vi "Voltage output module.vi"(0 "Device Select":string(combo)="None", 1 "Init":bool, 2 "Exec":bool, 3 "finish up":bool, 5 "Input Control pipe":T1, 7 "AO Channel":string(combo)="AO0", 11 "Error In":errorcluster, 12 "Voltage":dbl) -> (4 "current Control pipe":T1, 15 "Error out":errorcluster)   [LabVIEW 2023]
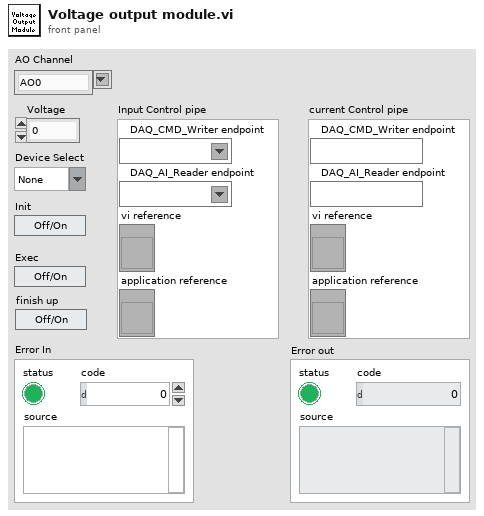
[diagram p1: front panel]
types:
  T1 = cluster{"DAQ_CMD_Writer endpoint":refnum<k21>, "DAQ_AI_Reader endpoint":refnum<k21>, "vi reference":refnum<vi>, "application reference":refnum<vi>}
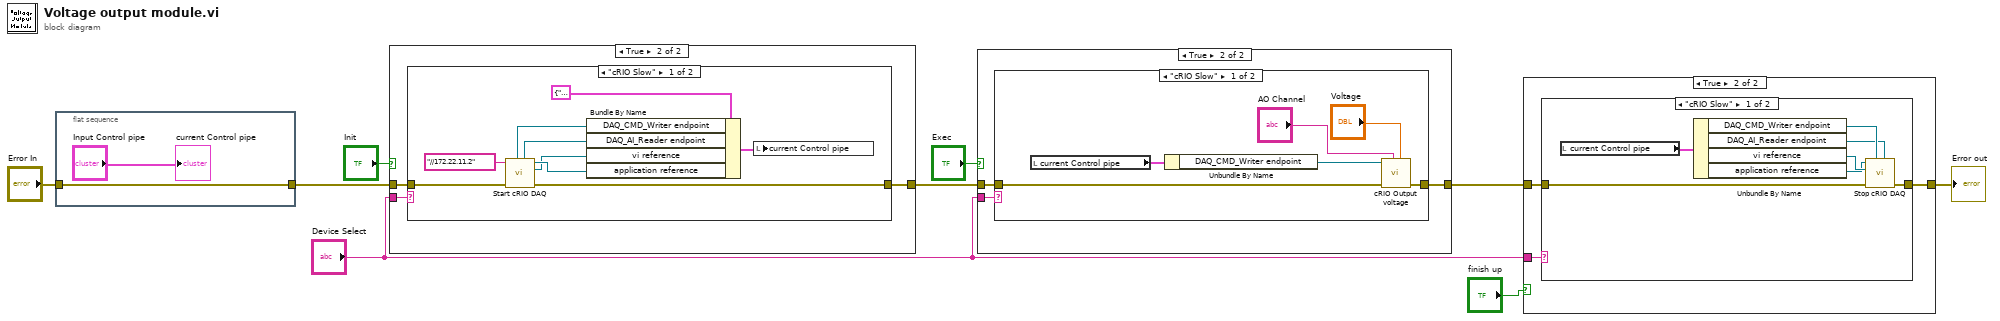
[diagram p0: block diagram]
diagram:
  n1 = flat-sequence {
    tunnel: "Error In" -> [w11]
    tunnel: [w11] -> w1
    frame #0 {
      "current Control pipe" <- "Input Control pipe"
    }
  }
  n2 = case shown="True" "Init" {
    tunnel: w1 -> [w12 w14]
    tunnel: [w12 w13] -> w6
    tunnel: "Device Select" -> [_ w15]
    frame False {
    }
    frame True {
      n3 = case shown="\"cRIO Slow\"" w15 {
        tunnel: w14 -> [w24 w25]
        tunnel: [w23 w25] -> w13
        frame "cRIO Slow" {
          n4 = call "Start cRIO DAQ.vi"("error in (no error)"=w24, "cRIO IP"="//172.22.11.2") -> ("error out"=w23:errorcluster, "vi reference"=w17:refnum<vi>, "application reference"=w18:refnum<vi>, "DAQ_AI_Reader endpoint"=w19:refnum<k21>, "DAQ_CMD_Writer endpoint"=w20:refnum<k21>)  [unwired: 5 in]
          n5 = Bundle By Name(cluster=T1 {"DAQ_CMD_Writer endpoint"="", "DAQ_AI_Reader endpoint"="", "vi reference"=refnum, "application reference"=refnum} ("current Control pipe"), "DAQ_CMD_Writer endpoint"=w20, "DAQ_AI_Reader endpoint"=w19, "vi reference"=w17, "application reference"=w18) -> (w16:T1)
          n6 = local write "current Control pipe"(w16) -> ()
        }
        frame "None", Default {
        }
      }
    }
  }
  n7 = case shown="True" "Exec" {
    tunnel: w6 -> [w26 w28]
    tunnel: [w26 w27] -> w5
    tunnel: "Device Select" -> [_ w29]
    frame False {
    }
    frame True {
      n8 = case shown="\"cRIO Slow\"" w29 {
        tunnel: w28 -> [w35 w36]
        tunnel: [w34 w36] -> w27
        frame "cRIO Slow" {
          n9 = local read "current Control pipe"() -> (w32:T1)
          n10 = Unbundle By Name(w32) -> ("DAQ_CMD_Writer endpoint"=w31:refnum<k21>)
          n11 = call "cRIO Output voltage.vi"("Voltage"="Voltage", "AO Channel"="AO Channel", "error in (no error)"=w35, "DAQ_CMD_Writer endpoint"=w31) -> ("error out"=w34:errorcluster)  [unwired: 6 in, 1 out]
        }
        frame "None", Default {
        }
      }
    }
  }
  n12 = case shown="True" "finish up" {
    tunnel: w5 -> [w37 w39]
    tunnel: [w37 w38] -> w4
    tunnel: "Device Select" -> [_ w40]
    frame False {
    }
    frame True {
      n13 = case shown="\"cRIO Slow\"" w40 {
        tunnel: w39 -> [w47 w48]
        tunnel: [w46 w48] -> w38
        frame "cRIO Slow" {
          n14 = local read "current Control pipe"() -> (w45:T1)
          n15 = Unbundle By Name(w45) -> ("DAQ_CMD_Writer endpoint"=w44:refnum<k21>, "DAQ_AI_Reader endpoint"=w43:refnum<k21>, "vi reference"=w42:refnum<vi>, "application reference"=w41:refnum<vi>)
          n16 = call "Stop cRIO DAQ.vi"("DAQ_AI_Reader endpoint"=w43, "DAQ_CMD_Writer endpoint"=w44, "error in (no error)"=w47, "VI reference"=w42, "application reference"=w41) -> ("error out"=w46:errorcluster)  [unwired: 6 in]
        }
        frame "None", Default {
        }
      }
    }
  }
  "Error out" <- w4
